vi "Buzzer.vi"   [LabVIEW 2020]
uses:
  <vilib>/sound2/lvsound2.llb/Sound Data Format.ctl
  <vilib>/sound2/lvsound2.llb/Sound Output Write (DBL).vi
types:
  T1 = typedef "Sound Data Format.ctl" = cluster{"sample rate (S/s)":dbl, "number of channels":i32, "bits per sample":i32}
  T2 = typedef "Sound Output Task ID.ctl" = u32
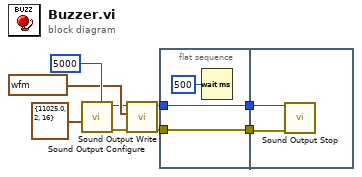
[diagram p0: block diagram]
diagram:
  n1 = call <vilib>:"Sound Output Configure.vi"("number of samples/ch"=5000, "sound format"=T1 {"sample rate (S/s)"=11025.0, "number of channels"=2, "bits per sample"=16}) -> ("error out"=w6:errorcluster, "task ID"=w7:T2)  [unwired: 8 in]
  n2 = call-poly <vilib>:"Sound Output Write.vi"("error in (no error)"=w6, "data"=waveform(dbl)[] [{"t0"=timestamp(0 s since 1904-01-01), "dt"=9.070294784580499e-05, "Y"=array[5000 elements]}] ("appended array"), "task ID"=w7) -> ("error out"=w3:errorcluster, "task ID out"=w4:T2)  [unwired: 7 in]
  n3 = flat-sequence {
    tunnel: w3 -> [w11]
    tunnel: w4 -> [w12]
    tunnel: [w12] -> w2
    tunnel: [w11] -> w1
    tunnel: w2 -> [w14]
    tunnel: w1 -> [w13]
    frame #0 {
      n4 = Wait (ms)(milliseconds to wait=u32 500) -> ()  [unwired: 1 out]
    }
    frame #1 {
      n5 = call <vilib>:"Sound Output Stop.vi"("error in (no error)"=w13, "task ID"=w14) -> ()  [unwired: 8 in, 2 out]
    }
  }
